vi "Get_operation.vi"(8 "error in (no error)":errorcluster, 11 "VISA resource in":refnum<visa-resource-name>) -> (0 "error out":errorcluster, 1 "CV":bool, 2 "CC":bool, 3 "VISA resource out":refnum<visa-resource-name>)   [LabVIEW 2014, in "B&K Precision 9120 series.lvclass"]
uses:
  B&K Precision 9120 series.lvclass
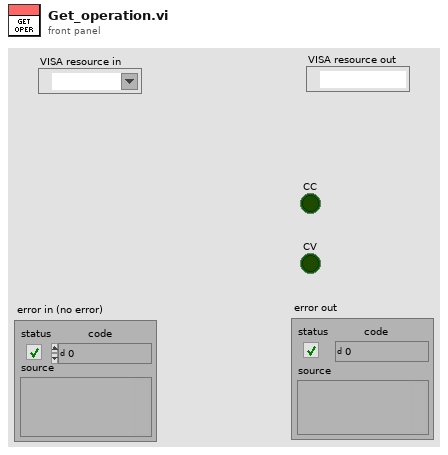
[diagram p1: front panel]
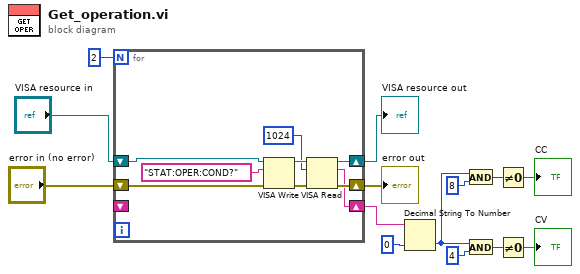
[diagram p0: block diagram]
diagram:
  n1 = for {
    N: 2 -> [_]
    shift-right: [w17] -> w11
    shift-left: "error in (no error)" -> [w23]
    shift-right: [w18] -> w12
    shift-left: "VISA resource in" -> [w22]
    shift-right: [w15] -> w10
    shift-left: _ -> [_]
    n2 = VISA Write(VISA resource name=w22, write buffer="STAT:OPER:COND?", error in (no error)=w23) -> (VISA resource name out=w21:refnum<visa-resource-name>, error out=w20:errorcluster)  [unwired: 1 out]
    n3 = VISA Read(VISA resource name=w21, byte count=u32 1024, error in (no error)=w20) -> (VISA resource name out=w18:refnum<visa-resource-name>, read buffer=w15:string, error out=w17:errorcluster)  [unwired: 1 out]
  }
  "VISA resource out" <- w12
  "error out" <- w11
  n4 = Decimal String To Number(string=w10, default (0L)=u32 0 ("default (0 DBL)")) -> (number=w6:u32)  [unwired: 1 in, 1 out]
  n5 = And(x=w6, y=u32 8) -> (x .and. y?=w8:u32)
  n6 = And(x=w6, y=u32 4) -> (x .and. y?=w5:u32)
  n7 = Not Equal To 0?(x=w8) -> (x != 0?=→"CC":bool)
  n8 = Not Equal To 0?(x=w5) -> (x != 0?=→"CV":bool)
